vi "example_insertSpace3.vi"() -> ()   [LabVIEW 2023]
uses:
  Ctrls/point.ctl
  BlockDiagram/BlockDiagram.lvclass
  C:/projects/TLC_Scripto/Source/AbstractDiagram/AbstractDiagram.lvclass
  TLC_Scripto.lvlib
  AbstractDiagram/AbstractDiagram.lvclass
panel:
  in  "origin":T1
  in  "deltaX":u16
  in  "deltaY":u16
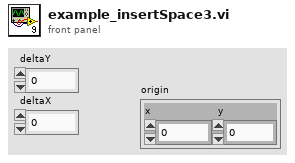
[diagram p1: front panel]
types:
  T1 = typedef "TLC_Scripto.lvlib/point.ctl" = cluster{"x":i32, "y":i32}
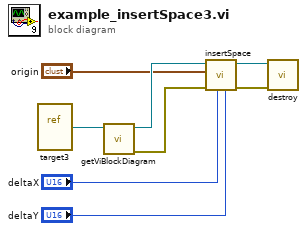
[diagram p0: block diagram]
diagram:
  n1 = vi-ref "target3.vi"() -> (w8:refnum<vi>)
  n2 = call "getViBlockDiagram.vi"("ViRef"=w8) -> ("error out"=w7:errorcluster, "topMostBlockDiagram"=w5:refnum<class "BlockDiagram.lvclass">)  [unwired: 9 in]
  n3 = call "insertSpace.vi"("deltaY"="deltaY", "deltaX"="deltaX", "error in (no error)"=w7, "origin"="origin", "AbstractDiagram In"=w5) -> ("error out"=w6:errorcluster, "AbstractDiagram Out"=w4:refnum<class "BlockDiagram.lvclass">)  [unwired: 5 in]
  n4 = call-dynamic "destroy.vi"("Error In"=w6, "Generic In"=w4) -> ()  [unwired: 9 in, 1 out]
